vi "MSScript_Format_LaserTrig.vi"(9 "ValueArray":string[](array[string]), 10 "TagArray":string[](array[string]), 11 "MSScript in":refnum<class "MSScript.lvclass">) -> (0 "ValueErrorArray":bool[](array[boolean]), 1 "TagErrorArray":bool[](array[boolean]), 2 "ParamErrorArray":bool[](array[boolean]), 3 "Data":variant, 4 "#ofParamError":bool)   [LabVIEW 2018, in "MSScript.lvclass"]
uses:
  MSScript.lvclass
  Ctl/MSEditorParam laserTrig.ctl
  MSScript_Transform_Extended.vi
  MSScript_Transform_UInt.vi
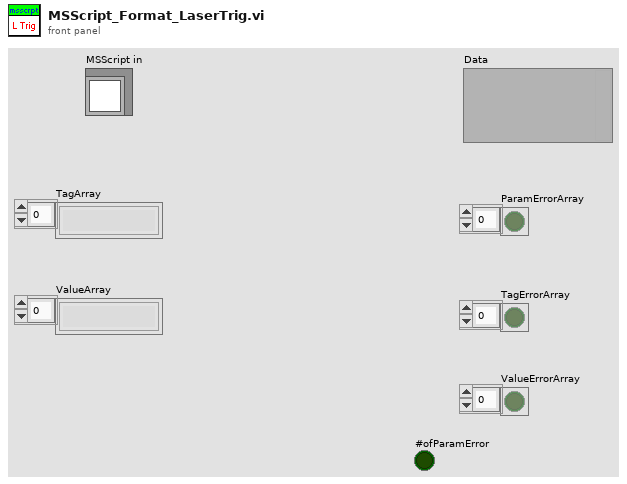
[diagram p1: front panel]
types:
  T1 = typedef "MSEditorParam laserTrig.ctl" = cluster{"trigFreq":ext, "phaseDeg":ext, "shots":u32}
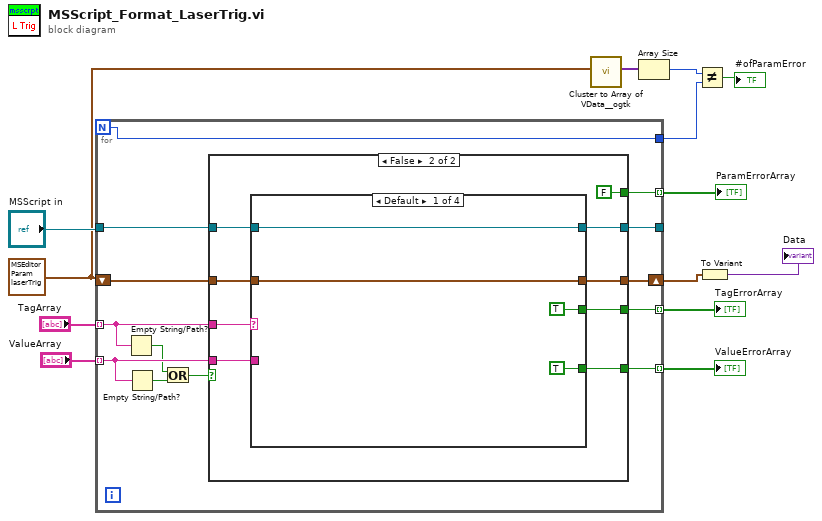
[diagram p0: block diagram]
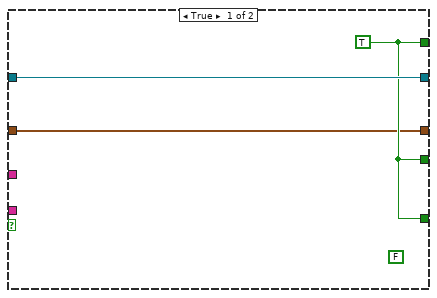
[diagram p2: hidden frame]
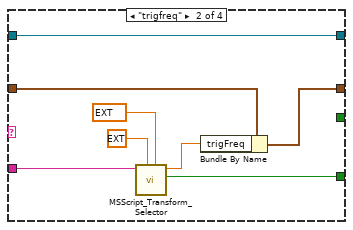
[diagram p3: hidden frame]
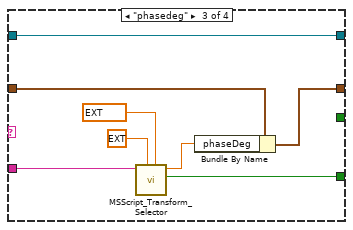
[diagram p4: hidden frame]
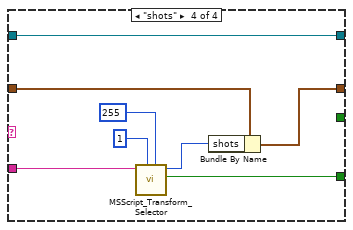
[diagram p5: hidden frame]
diagram:
  w4 = T1 {"trigFreq"=100.0, "phaseDeg"=90.0, "shots"=1} ("ParamValueType")
  n1 = for {
    N -> [w14]
    tunnel: "TagArray" -> [w22] mode=indexing
    tunnel: "ValueArray" -> [w21] mode=indexing
    tunnel: [w26] -> w11 mode=indexing
    tunnel: "MSScript in" -> [w25]
    tunnel: [w24] -> w10 mode=indexing
    tunnel: [w23] -> _
    tunnel: [w17] -> w9 mode=indexing
    shift-right: [w15] -> w2
    shift-left: w4 -> [w16]
    tunnel: [w14] -> w3
    n2 = Empty String/Path?(string/path=w22) -> (empty?=w19:bool)
    n3 = Empty String/Path?(string/path=w21) -> (empty?=w20:bool)
    n4 = Or(x=w19, y=w20) -> (x .or. y?=w18:bool)
    n5 = case shown="False" w18 {
      tunnel: [w28 w31] -> w26
      tunnel: w25 -> [w29 w34]
      tunnel: [w28 w30] -> w24
      tunnel: [w29 w33] -> w23
      tunnel: w22 -> [_ w36]
      tunnel: w21 -> [_ w37]
      tunnel: [w28 FALSE] -> w17
      tunnel: w16 -> [w27 w35]
      tunnel: [w27 w32] -> w15
      frame True {
        (unwired) FALSE ("Is a variable ?")
        w28 = TRUE
      }
      frame False {
        n6 = case shown="Default" w36 {
          tunnel: [TRUE _ _ _] -> w31
          tunnel: w34 -> [w40 w48 w56 w64]
          tunnel: w37 -> [_ w49 w57 w65]
          tunnel: [TRUE ("Value Error?") w50 w58 w66] -> w30
          tunnel: [w40 w48 w56 w64] -> w33
          tunnel: w35 -> [w39 w46 w54 w62]
          tunnel: [w39 w45 w53 w61] -> w32
          frame Default {
          }
          frame "trigfreq" {
            n7 = call-poly "MSScript_Transform_Selector.vi"("upper limit (Inf)"=ext 2000.0 ("upper limit"), "lower limit (-Inf)"=ext 1.0 ("lower limit"), "Check_Str"=w49) -> ("Value Error?"=w50:bool, "Value Output"=w47:ext)  [unwired: 6 in, 1 out]
            n8 = Bundle By Name(cluster=w46, "trigFreq"=w47) -> (w45:T1)
          }
          frame "phasedeg" {
            n9 = call-poly "MSScript_Transform_Selector.vi"("upper limit (Inf)"=ext 359.99 ("upper limit"), "lower limit (-Inf)"=ext 0.0 ("lower limit"), "Check_Str"=w57) -> ("Value Error?"=w58:bool, "Value Output"=w55:ext)  [unwired: 6 in, 1 out]
            n10 = Bundle By Name(cluster=w54, "phaseDeg"=w55) -> (w53:T1)
          }
          frame "shots" {
            n11 = call-poly "MSScript_Transform_Selector.vi"("upper limit"=u64 255, "lower limit"=u64 1, "string in"=w65) -> ("Value Error?"=w66:bool, "Value Output"=w63:u64)  [unwired: 6 in, 1 out]
            n12 = Bundle By Name(cluster=w62, "shots"=w63) -> (w61:T1)
          }
        }
      }
    }
  }
  "TagErrorArray" <- w11
  "ValueErrorArray" <- w10
  "ParamErrorArray" <- w9
  n13 = call <userlib>:"Cluster to Array of VData__ogtk.vi"("Cluster"=w4) -> ("Array of VData"=w7:variant[])  [unwired: 9 in, 1 out]
  n14 = Array Size(array=w7) -> (size(s)=w6:i32)
  n15 = Not Equal?(x=w6, y=w3) -> (x != y?=→"#ofParamError":bool)
  n16 = To Variant(anything=w2) -> (Variant=→"Data":variant)
